vi "json Parse I32 Array - array path.vi"(8 "error in (no error)":errorcluster, 9 "default":i32[](array[numeric]), 10 "path":string[](array[string]), 11 "JSON Document in":refnum<class "JSON Document.lvclass">) -> (0 "error out":errorcluster, 1 "defaulted?":bool, 2 "value":i32[](array[numeric]), 3 "JSON Document out":refnum<class "JSON Document.lvclass">, 4 "defaulted indices":i32[](array[numeric]))   [LabVIEW 2015, in "JSON Document.lvclass"]
uses:
  JSON Document.lvclass
  json Parse I32 Array - string path.vi
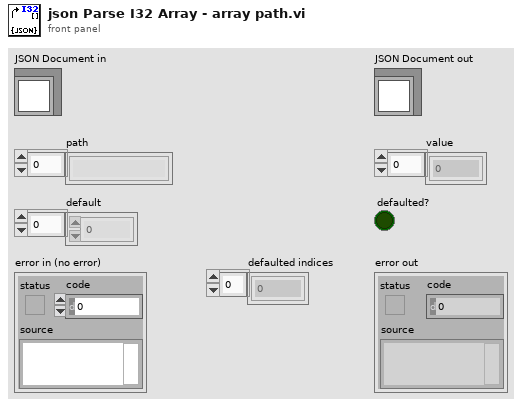
[diagram p1: front panel]
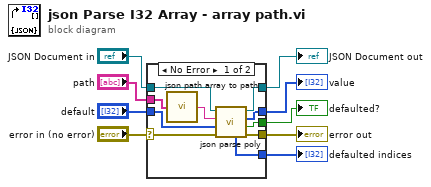
[diagram p0: block diagram]
diagram:
  n1 = case shown="No Error" "error in (no error)" {
    selector: "error in (no error)" -> [w16 w22]
    tunnel: [w11 w22] -> w8
    tunnel: [w13 w21] -> w6
    tunnel: "JSON Document in" -> [w19 w21]
    tunnel: "default" -> [w15 w20]
    tunnel: "path" -> [w18 _]
    tunnel: [w10 w20] -> w3
    tunnel: [w14 _] -> w2
    tunnel: [w12 _] -> w1
    frame No Error {
      n2 = call "json path array to path.vi"("path"=w18) -> ("String"=w17:string)
      n3 = call-poly "json parse poly.vi"("error in (no error)"=w16, "default"=w15, "path"=w17, "JSON Document in"=w19) -> ("error out"=w11:errorcluster, "defaulted?"=w14:bool, "value"=w10:i32[], "JSON Document out"=w13:refnum<class "JSON Document.lvclass">, "defaulted indices"=w12:i32[])  [unwired: 3 in]
    }
    frame Error {
    }
  }
  "error out" <- w8
  "JSON Document out" <- w6
  "value" <- w3
  "defaulted?" <- w2
  "defaulted indices" <- w1
